vi "Configure Modulation (Phase).vi"(0 "VISA resource name":refnum<visa-resource-name>, 1 "Enable PM (T:Enable)":bool=TRUE, 2 "PM Path (1)":u16(ring)=1 items=["1"=1, "2"=2], 5 "Enable Deviation Coupling (T:Enable)":bool=TRUE, 7 "PM Deviation (0 rad)":dbl, 9 "Phase Bandwidth (0: Normal)":u16(ring) items=["Normal", "High"], 11 "error in (no error)":errorcluster) -> (4 "VISA resource name out":refnum<visa-resource-name>, 15 "error out":errorcluster)   [LabVIEW 2009, in "Agilent PSG MXG Series.lvlib"]
doc: "Configures phase modulation.\n\n<B>Notes:</B>\n(1) This VI is <B>NOT</B> valid in E8247C.\n\n(2) For E8257D, E8267D, N5181A, N5182A, N5183A, this VI is valid only when the instument installs <B>Option UNT</B> (AM, FM, phase modulation)."
uses:
  Agilent PSG MXG Series.lvlib
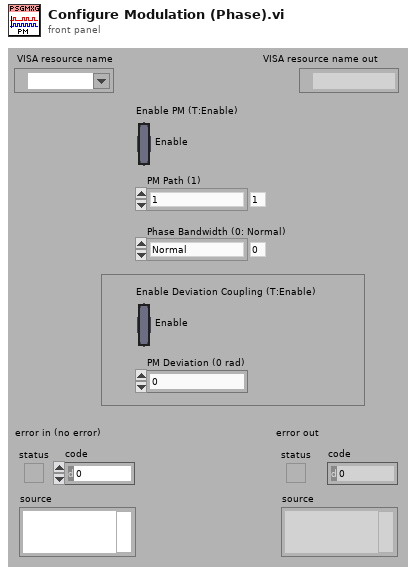
[diagram p1: front panel]
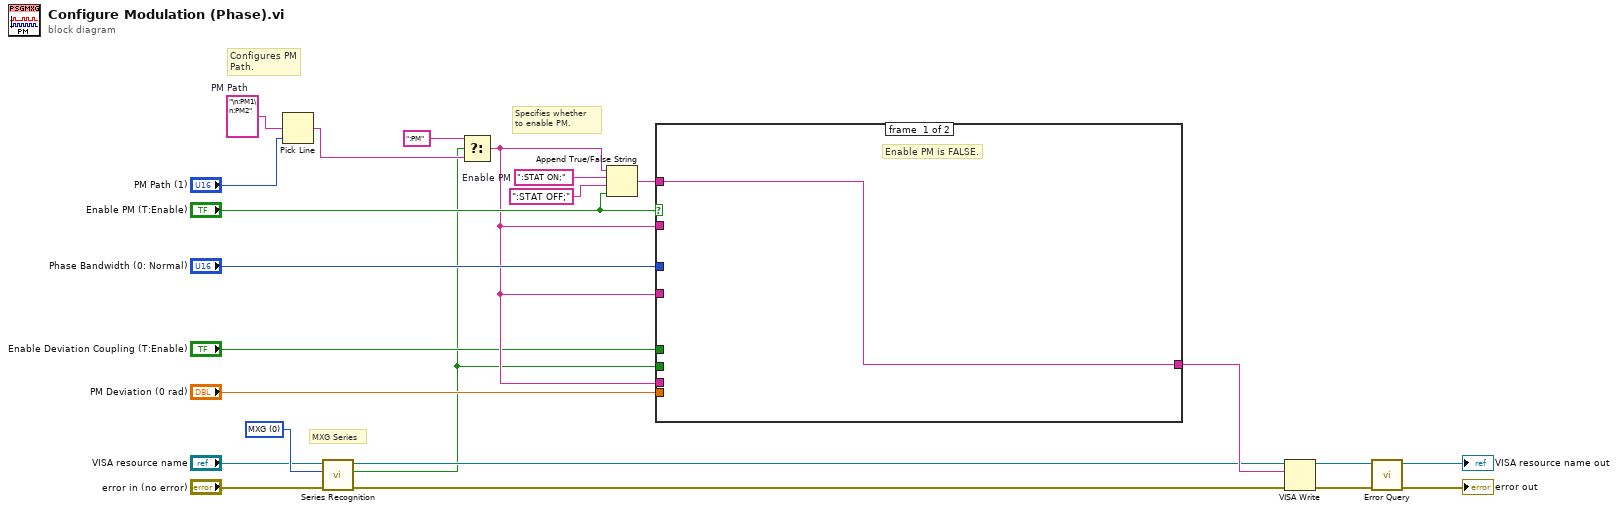
[diagram p0: block diagram]
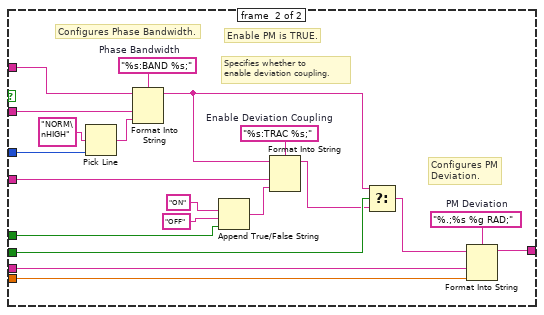
[diagram p2: hidden frame]
diagram:
  w6 = u16 0 items=["MXG", "PSG", "PSG-A", "PSG-C", "PSG-D"] ("Series Type (0: MXG)")
  w20 = ":STAT ON;"  # Enable PM
  w23 = "\n:PM1\n:PM2"  # PM Path
  # "Specifies whether\nto enable PM."
  # "Configures PM\nPath."
  # "MXG Series"
  n1 = Pick Line(multi-line string=w23, line index="PM Path (1)") -> (output string=w22:string)  [unwired: 1 out]
  n2 = call "Series Recognition.vi"("error in (no error)"="error in (no error)", "Series Type (0: MXG)"=w6, "VISA resource name"="VISA resource name") -> ("error out"=w7:errorcluster, "Is Series Correct"=w5:bool, "VISA resource name out"=w8:refnum<visa-resource-name>)  [unwired: 6 out]
  n3 = Select(t=":PM", s=w5, f=w22) -> (s? t:f=w11:string)
  n4 = Append True/False String(1:"Enable PM (T:Enable)", 2:":STAT OFF;" ("true string"), 3:w20, 4:w11) -> (0:w16:string)
  n5 = case shown="True" "Enable PM (T:Enable)" {
    tunnel: w11 -> [_ w43]
    tunnel: "Enable Deviation Coupling (T:Enable)" -> [_ w40]
    tunnel: w5 -> [_ w39]
    tunnel: w16 -> [w24 w31]
    tunnel: w11 -> [_ w35]
    tunnel: "PM Deviation (0 rad)" -> [_ w34]
    tunnel: [w24 w33] -> w15
    tunnel: "Phase Bandwidth (0: Normal)" -> [_ w28]
    tunnel: w11 -> [_ w27]
    frame #0 {
      # "Enable PM is FALSE."
    }
    frame #1 {
      w32 = "%s:BAND %s;"  # Phase Bandwidth
      w37 = "%.;%s %g RAD;"  # PM Deviation
      w44 = "%s:TRAC %s;"  # Enable Deviation Coupling
      # "Configures PM\nDeviation."
      # "Specifies whether to\nenable deviation coupling."
      # "Configures Phase Bandwidth."
      # "Enable PM is TRUE."
      n6 = Pick Line(multi-line string="NORM\nHIGH", line index=w28) -> (output string=w30:string)  [unwired: 1 out]
      n7 = Format Into String(format string=w32, initial string=w31, w27, w30) -> (resulting string=w26:string)  [unwired: 1 in, 1 out]
      n8 = Append True/False String(1:w40, 2:"OFF" ("false string"), 3:"ON" ("true string")) -> (0:w42:string)  [unwired: 1 out]
      n9 = Format Into String(format string=w44, initial string=w26, w43, w42) -> (resulting string=w38:string)  [unwired: 1 in, 1 out]
      n10 = Select(t=w26, s=w39, f=w38) -> (s? t:f=w36:string)
      n11 = Format Into String(format string=w37, initial string=w36, w35, w34) -> (resulting string=w33:string)  [unwired: 1 in, 1 out]
    }
  }
  n12 = VISA Write(VISA resource name=w8, write buffer=w15, error in (no error)=w7) -> (VISA resource name out=w18:refnum<visa-resource-name>, error out=w17:errorcluster)  [unwired: 1 out]
  n13 = call "Error Query.vi"("error in (no error)"=w17, "VISA resource name"=w18) -> ("error out"=→"error out":errorcluster, "VISA resource name out"=→"VISA resource name out":refnum<visa-resource-name>)  [unwired: 8 out]
